vi "Shutdown_button.vi"() -> ()   [LabVIEW 2018]
uses:
  <vilib>/userdefined/High Color/nirio_resource_hc.ctl
  <vilib>/FPGAPlugInAG/PXI-7951R/niLvFpga_Open_PXI-7951R.vi
  <vilib>/FPGAPlugInAG/PXI-7951R/niLvFpga_Reset_PXI-7951R.vi
  <vilib>/FPGAPlugInAG/PXI-7951R/niLvFpga_Run_PXI-7951R.vi
  <vilib>/Utility/error.llb/Error Cluster From Error Code.vi
  <vilib>/rvi/errors/niLvFpgaAdjustHostInterfaceError.vi
  <vilib>/FPGAPlugInAG/PXI-7951R/niLvFpga_Close_PXI-7951R.vi
  <vilib>/rvi/interface/nirviOpenFPGA/nirviOpenFPGA.xnode
  FPGA Bitfiles/StudyFPGA_FPGATarget_Miganie_yjd+di0icDE.lvbitx
  <vilib>/rvi/interface/nirviMethod/nirviMethod.xnode
  <vilib>/rvi/interface/nirviReadWriteControl/nirviReadWriteControl.xnode
  <vilib>/rvi/interface/nirviCloseFPGA/nirviCloseFPGA.xnode
  NiFpgaLv.dll
panel:
  in  "0.7":bool
  in  "0.6":bool
  in  "0.5":bool
  in  "0.4":bool
  in  "0.3":bool
  in  "0.2":bool
  in  "0.1":bool
  in  "0.0":bool
  out "IO Module\\DDCB_Port2_Read":u8 format="%b"
  out "IO Module\\DDCB_Port1_Read":u8 format="%b"
  out "IO Module\\DDCB_Port0_Read":u8 format="%b"
  out "IO Module\\DDCA_Port2_Read":u8 format="%b"
  out "IO Module\\DDCA_Port1_Read":u8 format="%b"
  in  "Current limit CH1":dbl=0.1 format="%#_13g"
  in  "Current limit CH2":dbl=0.1 format="%#_13g"
  in  "Stop Power":bool
  in  "Voltage level CH0":dbl=3.0 format="%#_13g"
  in  "Output enabled CH0":bool
  in  "Voltage level CH1":dbl=3.0 format="%#_13g"
  in  "Voltage level CH2":dbl=-1.0 format="%#_13g"
  in  "Output enabled CH2":bool
  in  "Output enabled CH1":bool
  in  "Current limit CH0":dbl=0.1 format="%#_13g"
  in  "Power Resource":refnum<k15>="PXI1Slot3"
  out "IO Module\\DDCA_Port0_Read":u8 format="%b"
  out "error out":errorcluster
  in  "resource name":T1="PXI1Slot2" caption="RIO Device"
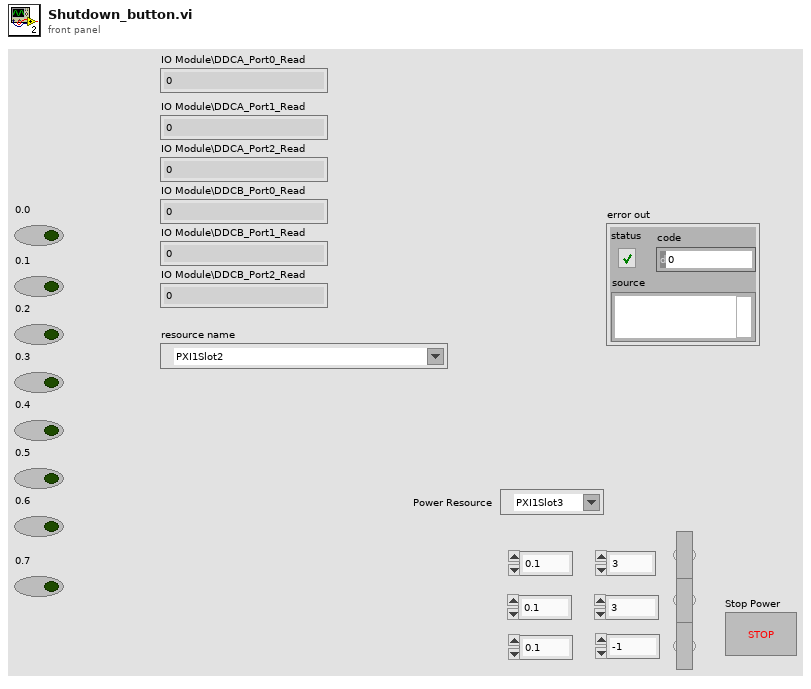
[diagram p1: front panel]
types:
  T1 = typedef "nirio_resource_hc.ctl" = tag
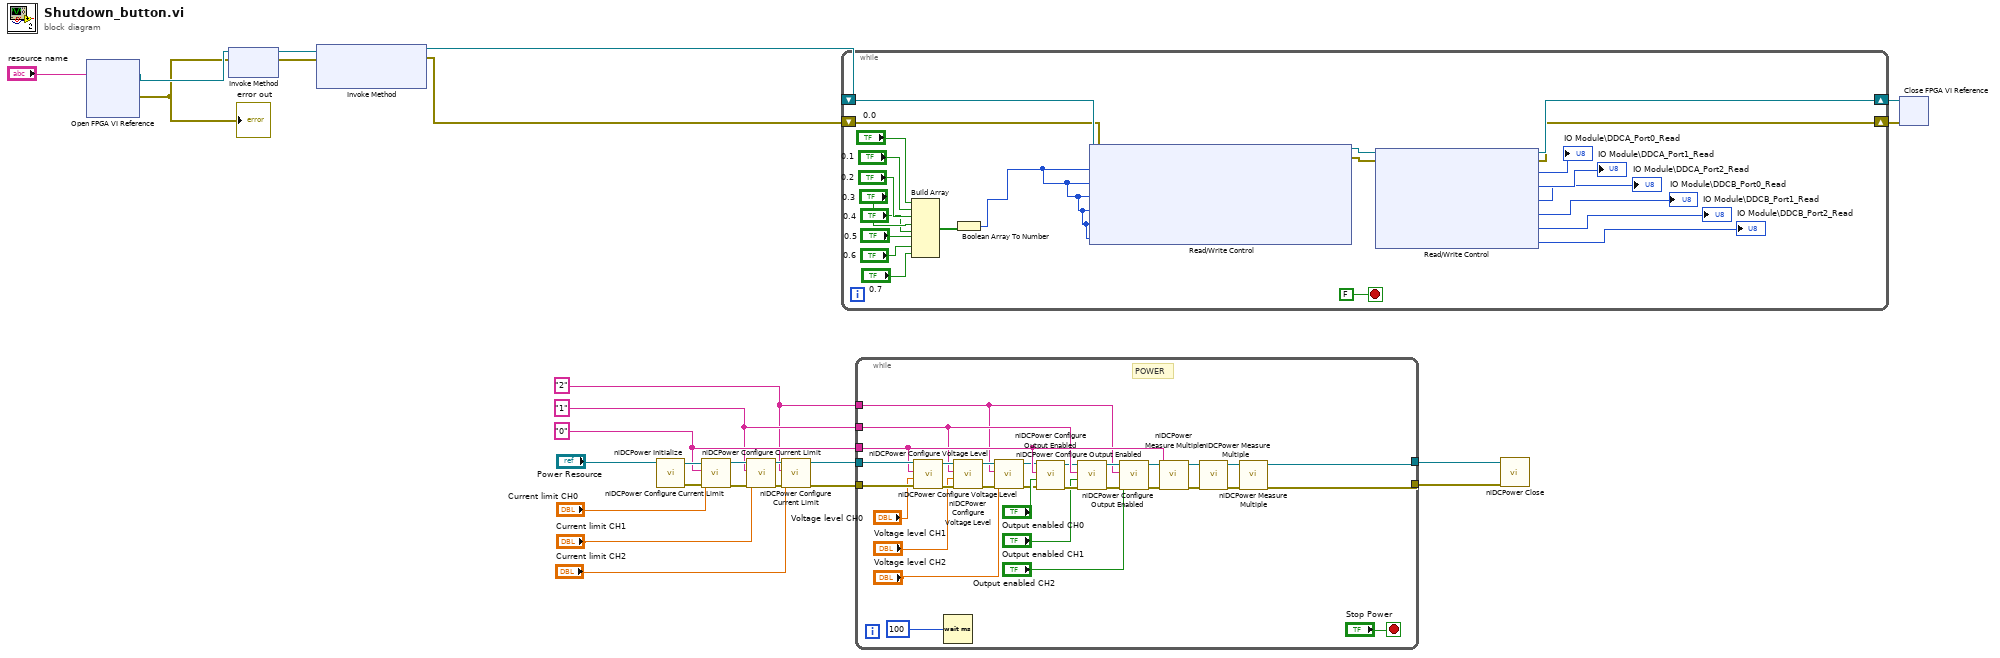
[diagram p0: block diagram]
diagram:
  w2 = "2"
  w3 = "1"
  w11 = "0" ("Channel name")
  n1 = xnode "Open FPGA VI Reference"("resource name"="resource name") -> ("FPGA VI Reference Out"=w25:refnum<k20>, "error out"=w24:errorcluster)  [unwired: 1 in]
  "error out" <- w24
  n2 = xnode "Invoke Method"("FPGA VI Reference In"=w25, "error in"=w24) -> ("FPGA VI Reference Out"=w19:refnum<k20>, "error out"=w18:errorcluster)
  n3 = xnode ("Invoke Method")("FPGA VI Reference In"=w19, "error in"=w18) -> ("FPGA VI Reference Out"=w21:refnum<k20>, "error out"=w20:errorcluster)  [unwired: 1 in]
  n4 = call <instrlib>:"niDCPower Initialize.vi"("resource name"="Power Resource") -> ("error out"=w14:errorcluster, "instrument handle out"=w15:refnum<k15>)  [unwired: 3 in, 6 out]
  n5 = call <instrlib>:"niDCPower Configure Current Limit.vi"("error in (no error)"=w14, "current limit"="Current limit CH0", "channel name"=w11, "instrument handle"=w15) -> ("error out"=w7:errorcluster, "instrument handle out"=w10:refnum<k15>)  [unwired: 6 in]
  n6 = call <instrlib>:"niDCPower Configure Current Limit.vi"("error in (no error)"=w7, "current limit"="Current limit CH1", "channel name"=w3, "instrument handle"=w10) -> ("error out"=w6:errorcluster, "instrument handle out"=w9:refnum<k15>)  [unwired: 6 in]
  n7 = call <instrlib>:"niDCPower Configure Current Limit.vi"("error in (no error)"=w6, "current limit"="Current limit CH2", "channel name"=w2, "instrument handle"=w9) -> ("error out"=w5:errorcluster, "instrument handle out"=w8:refnum<k15>)  [unwired: 6 in]
  n8 = while {
    shift-right: [w44] -> w23
    shift-left: w21 -> [w49]
    shift-right: [w43] -> w22
    shift-left: w20 -> [w48]
    stop <- FALSE stop-if-true
    n9 = Build Array("0.0", "0.1", "0.2", "0.3", "0.4", "0.5", "0.6", "0.7") -> (w28:bool[])
    n10 = Boolean Array To Number(Boolean array=w28) -> (number=w27:u32)
    n11 = xnode "Read/Write Control"("FPGA VI Reference In"=w49, "error in"=w48, "IO Module\\DDCA_Port0_Write"=w27, "IO Module\\DDCA_Port1_Write"=w27, "IO Module\\DDCA_Port2_Write"=w27, "IO Module\\DDCB_Port0_Write"=w27, "IO Module\\DDCB_Port1_Write"=w27, "IO Module\\DDCB_Port2_Write"=w27) -> ("FPGA VI Reference Out"=w46:refnum<k20>, "error out"=w45:errorcluster)
    n12 = xnode "Read/Write Control"("FPGA VI Reference In"=w46, "error in"=w45) -> ("FPGA VI Reference Out"=w44:refnum<k20>, "error out"=w43:errorcluster, "IO Module\\DDCA_Port0_Read"=→"IO Module\\DDCA_Port0_Read":u8, "IO Module\\DDCA_Port1_Read"=→"IO Module\\DDCA_Port1_Read":u8, "IO Module\\DDCA_Port2_Read"=→"IO Module\\DDCA_Port2_Read":u8, "IO Module\\DDCB_Port0_Read"=→"IO Module\\DDCB_Port0_Read":u8, "IO Module\\DDCB_Port1_Read"=→"IO Module\\DDCB_Port1_Read":u8, "IO Module\\DDCB_Port2_Read"=→"IO Module\\DDCB_Port2_Read":u8)
  }
  n13 = while {
    tunnel: w11 -> [w74]
    tunnel: [w53] -> w13
    tunnel: [w56] -> w12
    tunnel: w5 -> [w79]
    tunnel: w8 -> [w78]
    tunnel: w3 -> [w66]
    tunnel: w2 -> [w61]
    stop <- "Stop Power" stop-if-true
    # "POWER"
    n14 = call <instrlib>:"niDCPower Configure Voltage Level.vi"("error in (no error)"=w79, "voltage level"="Voltage level CH0", "channel name"=w74, "instrument handle"=w78) -> ("error out"=w73:errorcluster, "instrument handle out"=w68:refnum<k15>)  [unwired: 6 in]
    n15 = Wait (ms)(milliseconds to wait=u32 100) -> ()  [unwired: 1 out]
    n16 = call <instrlib>:"niDCPower Configure Voltage Level.vi"("error in (no error)"=w73, "voltage level"="Voltage level CH1", "channel name"=w66, "instrument handle"=w68) -> ("error out"=w72:errorcluster, "instrument handle out"=w67:refnum<k15>)  [unwired: 6 in]
    n17 = call <instrlib>:"niDCPower Configure Voltage Level.vi"("error in (no error)"=w72, "voltage level"="Voltage level CH2", "channel name"=w61, "instrument handle"=w67) -> ("error out"=w70:errorcluster, "instrument handle out"=w69:refnum<k15>)  [unwired: 6 in]
    n18 = call <instrlib>:"niDCPower Configure Output Enabled.vi"("error in (no error)"=w70, "output enabled"="Output enabled CH0", "channel name"=w74, "instrument handle"=w69) -> ("error out"=w64:errorcluster, "instrument handle out"=w65:refnum<k15>)  [unwired: 6 in]
    n19 = call <instrlib>:"niDCPower Configure Output Enabled.vi"("error in (no error)"=w64, "output enabled"="Output enabled CH1", "channel name"=w66, "instrument handle"=w65) -> ("error out"=w63:errorcluster, "instrument handle out"=w62:refnum<k15>)  [unwired: 6 in]
    n20 = call <instrlib>:"niDCPower Configure Output Enabled.vi"("error in (no error)"=w63, "output enabled"="Output enabled CH2", "channel name"=w61, "instrument handle"=w62) -> ("error out"=w59:errorcluster, "instrument handle out"=w60:refnum<k15>)  [unwired: 6 in]
    n21 = call <instrlib>:"niDCPower Measure Multiple.vi"("error in (no error)"=w59, "channel name"=w74, "instrument handle"=w60) -> ("error out"=w55:errorcluster, "instrument handle out"=w58:refnum<k15>)  [unwired: 5 in, 2 out]
    n22 = call <instrlib>:"niDCPower Measure Multiple.vi"("error in (no error)"=w55, "instrument handle"=w58) -> ("error out"=w54:errorcluster, "instrument handle out"=w57:refnum<k15>)  [unwired: 6 in, 2 out]
    n23 = call <instrlib>:"niDCPower Measure Multiple.vi"("error in (no error)"=w54, "instrument handle"=w57) -> ("error out"=w53:errorcluster, "instrument handle out"=w56:refnum<k15>)  [unwired: 6 in, 2 out]
  }
  n24 = call <instrlib>:"niDCPower Close.vi"("error in (no error)"=w13, "instrument handle"=w12) -> ()  [unwired: 9 in, 1 out]
  n25 = xnode "Close FPGA VI Reference"("FPGA VI Reference In"=w23, "error in"=w22) -> ()  [unwired: 1 out]
